vi "OICB - Get Analog.vi"(8 "error in (no error)":errorcluster) -> (0 "error out":errorcluster, 3 "Analog":T1)   [LabVIEW 2015]
uses:
  Analog_Input_TypeDef.ctl
  <vilib>/Rock Robotics/Network Tables/NT Read String.vi
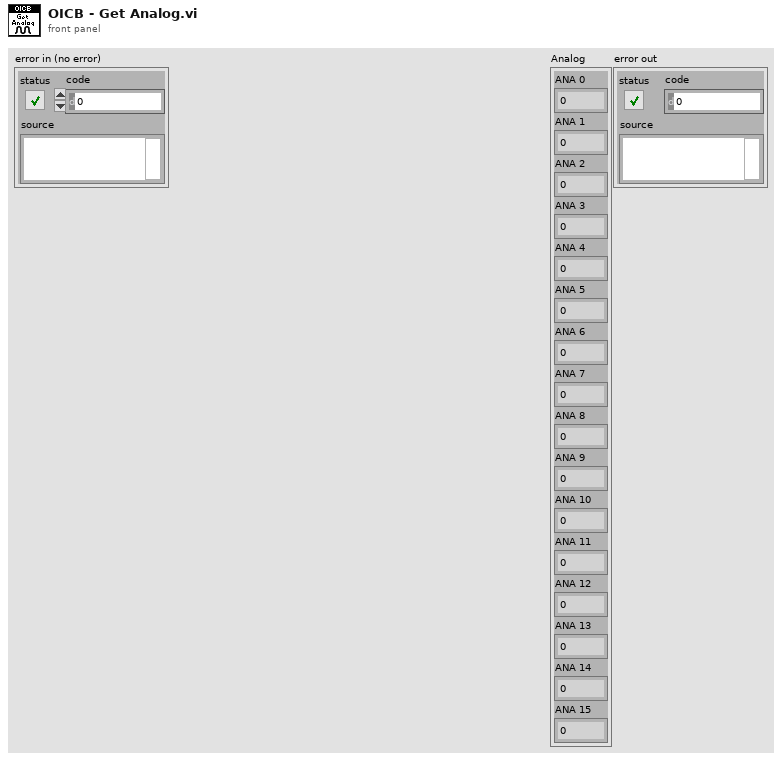
[diagram p1: front panel]
types:
  T1 = typedef "Analog_Input_TypeDef.ctl" = cluster{"ANA 0":u8, "ANA 1":u8, "ANA 2":u8, "ANA 3":u8, "ANA 4":u8, "ANA 5":u8, "ANA 6":u8, "ANA 7":u8, "ANA 8":u8, "ANA 9":u8, "ANA 10":u8, "ANA 11":u8, "ANA 12":u8, "ANA 13":u8, "ANA 14":u8, "ANA 15":u8}
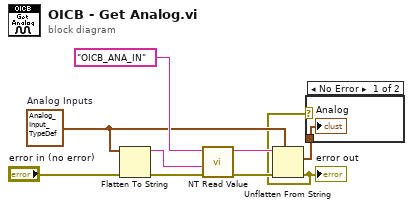
[diagram p0: block diagram]
diagram:
  w8 = T1 {"ANA 0"=0, "ANA 1"=0, "ANA 2"=0, "ANA 3"=0, "ANA 4"=0, "ANA 5"=0, "ANA 6"=0, "ANA 7"=0, "ANA 8"=0, "ANA 9"=0, "ANA 10"=0, "ANA 11"=0, "ANA 12"=0, "ANA 13"=0, "ANA 14"=0, "ANA 15"=0}  # Analog Inputs
  n1 = Flatten To String(anything=w8, error in (no error)="error in (no error)") -> (data string=w6:string, error out=w7:errorcluster)  [unwired: 2 in, 1 out]
  n2 = call-poly <vilib>:"NT Read Value.vi"("error in"=w7, "Default Value"=w6, "Name"="OICB_ANA_IN") -> ("error out"=w5:errorcluster, "String"=w4:string)  [unwired: 7 in]
  n3 = Unflatten From String(type=w8, binary string=w4, error in (no error)=w5) -> (value=w3:T1, error out=w1:errorcluster)  [unwired: 2 in, 1 out]
  "error out" <- w1
  n4 = case shown="No Error" w1 {
    tunnel: w3 -> [w10 _]
    frame No Error {
      "Analog" <- w10
    }
    frame Error {
    }
  }
